vi "Demo.vi"() -> ()   [LabVIEW 2019]
uses:
  Components/MES_Base.lvlibp/Controls/Test.ctl
  Components/TestView_Base.lvlibp/ViewStatus.ctl
  Components/TestView_Base.lvlibp/TestView_Base.lvclass
  C:/Projects/Client-Nanosonics/Src/Components/ViPER.lvlibp/ViPER.lvclass
  Components/ViPER.lvlibp/ViPER.lvclass
  Components/MES_Base.lvlibp/MES_Base.lvclass
panel:
  in  "Exit":bool caption="Blank"
  out "error out":errorcluster
  in  "Clear":bool
  in  "DUT":u32
  in  "User":string
  in  "set User":bool
  in  "Status":T1
  in  "set status":bool
  in  "Test":T2={"Code"="", "Name"="", "Description"="", "Group"="", "IsGroup"=FALSE, "Tag"="", "Method"="", "Parrameter"="", "DataType"=enum."String", "Value"=variant, "Status"=enum."Pass", "LimitLo"=variant, "LimitHi"=variant, "StringMatch"="", "BooleanMatch"=FALSE, "DisplayFormat"="", "Units"="", "TestTime"=0.0}
  in  "Set test":bool
  in  "Tests":T2[](array[typedef])
  in  "Set tests":bool
  in  "Title":string
  in  "set title":bool
  in  "SN":string
  in  "set SN":bool
  in  "stop":bool
  in  "Config XML":string="<?xml version=\"1.0\" encoding=\"UTF-8\" standalone=\"no\" ?>\n<Object>\n\n  <Name>TestView</Name>\n\n  <Class>TestView_Bailey</Class>\n\n</Object>\n"
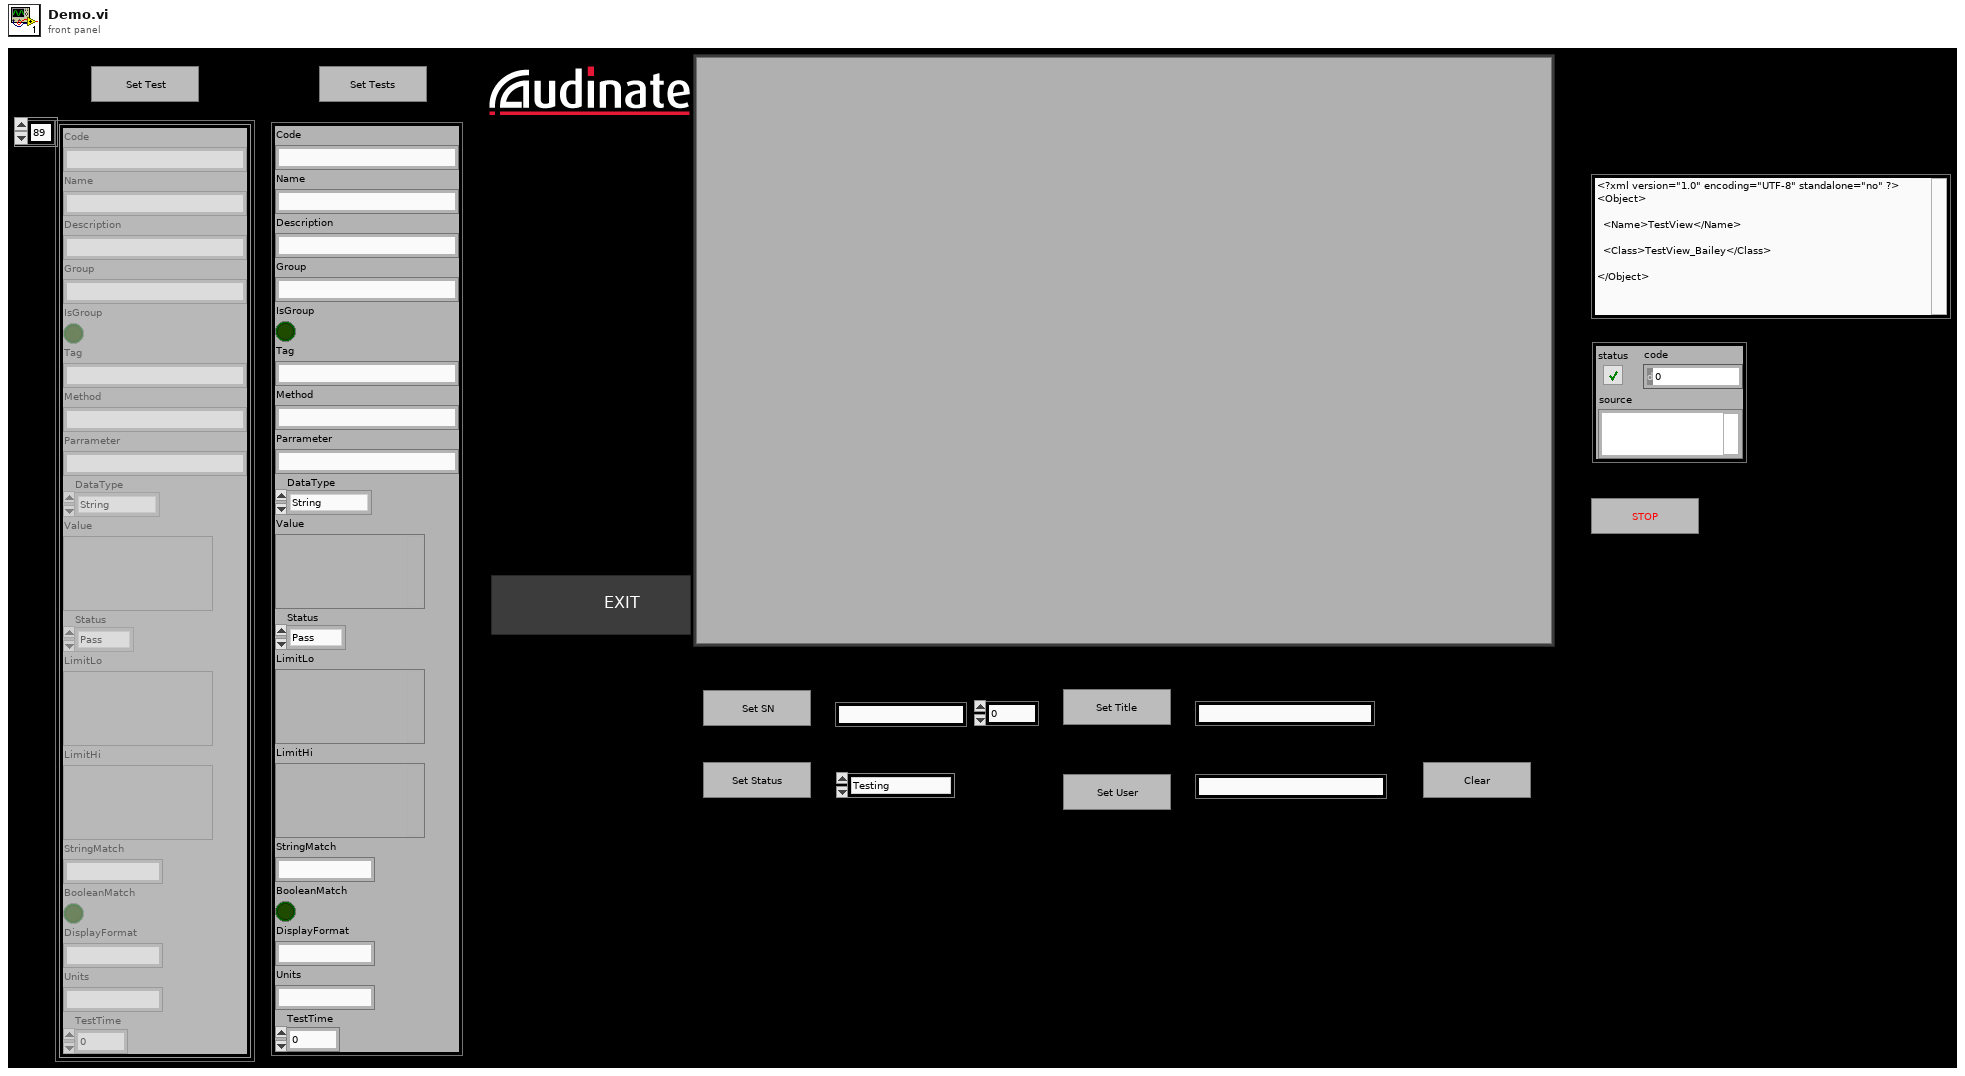
[diagram p1: front panel]
types:
  T1 = typedef "TestView_Base.lvlibp/TestView_Base.lvclass/ViewStatus.ctl" = enum16{"Testing", "Ready", "Logout", "Login", "PASS", "FAIL", "FAULT", "ABORTED"}
  T2 = typedef "MES_Base.lvlibp/MES_Base.lvclass/Test.ctl" = cluster{"Code":string, "Name":string, "Description":string, "Group":string, "IsGroup":bool, "Tag":string, "Method":string, "Parrameter":string, "DataType":enum16{"NA", "String", "Boolean", "Int", "Dbl"}, "Value":variant, "Status":enum16{"Pending", "Pass", "Fail"}, "LimitLo":variant, "LimitHi":variant, "StringMatch":string, "BooleanMatch":bool, "DisplayFormat":string, "Units":string, "TestTime":dbl}
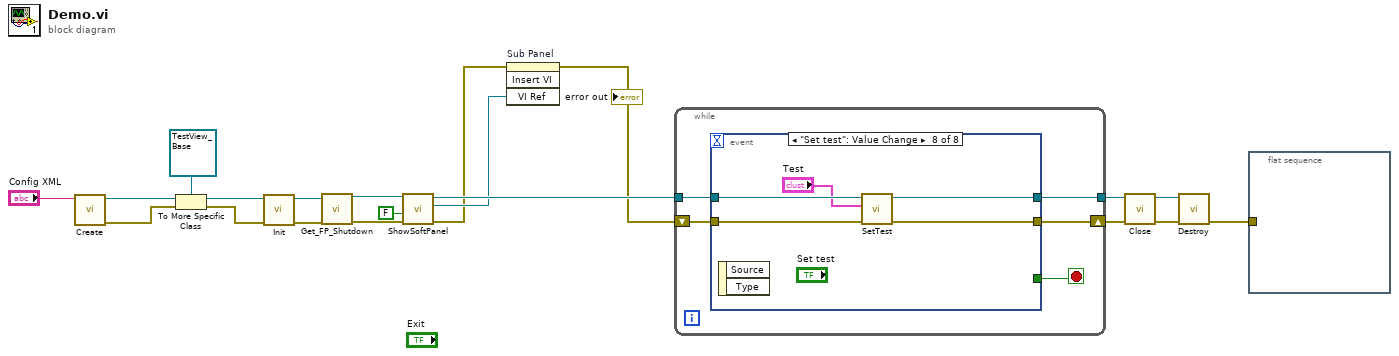
[diagram p0: block diagram]
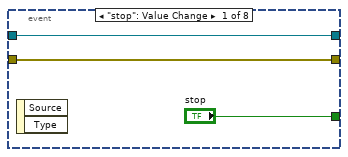
[diagram p2: hidden frame]
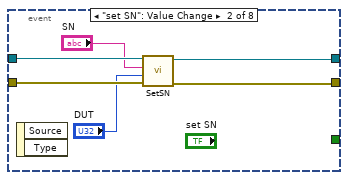
[diagram p3: hidden frame]
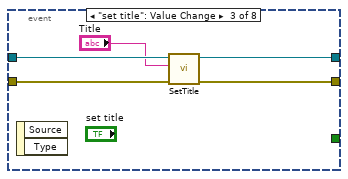
[diagram p4: hidden frame]
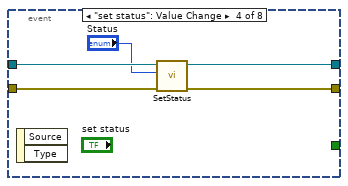
[diagram p5: hidden frame]
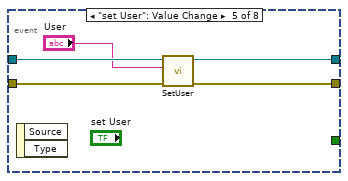
[diagram p6: hidden frame]
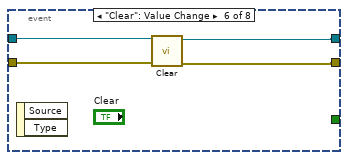
[diagram p7: hidden frame]
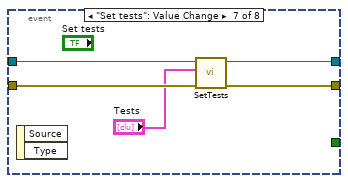
[diagram p8: hidden frame]
diagram:
  n1 = call "Create.vi"("Config XML"="Config XML") -> ("error out"=w9:errorcluster, "reference out"=w7:refnum<class "ViPER.lvclass">)  [unwired: 9 in]
  n2 = To More Specific Class(target class=refnum<class "TestView_Base.lvclass"> refnum ("TestView_Base.lvlibp:TestView_Tree"), reference=w7, error in=w9) -> (specific class reference=w6:refnum<class "TestView_Base.lvclass">, error out=w8:errorcluster)
  n3 = call-dynamic "Init.vi"("error in (no error)"=w8, "reference in"=w6) -> ("error out"=w19:errorcluster, "reference in"=w18:refnum<class "TestView_Base.lvclass">)  [unwired: 8 in]
  n4 = call "Get_FP_Shutdown.vi"("ViKing_Base in"=w18, "error in (no error)"=w19) -> ("ViKing_Base out"=w16:refnum<class "TestView_Base.lvclass">, "error out"=w17:errorcluster)  [unwired: 9 in, 3 out]
  n5 = call-dynamic "ShowSoftPanel.vi"("error in (no error)"=w17, "Floating"=FALSE, "Driver in"=w16) -> ("error out"=w2:errorcluster, "vi reference"=w3:refnum<vi>, "Driver out"=w5:refnum<class "TestView_Base.lvclass">)  [unwired: 6 in]
  n6 = invoke on="Sub Panel" class="SubPnl" method="Insert VI"(error in=w2, "VI Ref"=w3) -> (error out=w1:errorcluster)  [unwired: 2 in, 3 out]
  "error out" <- w1
  n7 = while {
    tunnel: w5 -> [w24]
    shift-right: [w22] -> w12
    shift-left: w1 -> [w25]
    tunnel: [w21] -> w13
    stop <- w23 stop-if-true
    n8 = event shown="[7] \"Set test\": Value Change" {
      selector: _ -> [_ _ _ _ _ _ _ _]
      dyn-events: _ -> [_ _ _ _ _ _ _ _]
      timeout: _ -> [_ _ _ _ _ _ _ _]
      tunnel: w25 -> [w27 w34 w39 w44 w49 w53 w58 w63]
      tunnel: w24 -> [w26 w33 w38 w43 w48 w52 w56 w62]
      tunnel: ["stop" _ _ _ _ _ _ _] -> w23
      tunnel: [w27 w32 w37 w42 w47 w51 w57 w61] -> w22
      tunnel: [w26 w31 w36 w41 w46 w50 w55 w60] -> w21
      event "stop": Value Change {
        n9 = event-data() -> ()  [unwired: 1 in, 2 out]
      }
      event "set SN": Value Change {
        n10 = event-data() -> ()  [unwired: 1 in, 2 out]
        n11 = call-dynamic "SetSN.vi"("error in (no error)"=w34, "DUT"="DUT", "SN"="SN", "reference in"=w33) -> ("error out"=w32:errorcluster, "reference in"=w31:refnum<class "TestView_Base.lvclass">)  [unwired: 6 in]
      }
      event "set title": Value Change {
        n12 = event-data() -> ()  [unwired: 1 in, 2 out]
        n13 = call-dynamic "SetTitle.vi"("error in (no error)"=w39, "Title"="Title", "reference in"=w38) -> ("error out"=w37:errorcluster, "reference in"=w36:refnum<class "TestView_Base.lvclass">)  [unwired: 7 in]
      }
      event "set status": Value Change {
        n14 = event-data() -> ()  [unwired: 1 in, 2 out]
        n15 = call-dynamic "SetStatus.vi"("error in (no error)"=w44, "Status"="Status", "reference in"=w43) -> ("error out"=w42:errorcluster, "reference in"=w41:refnum<class "TestView_Base.lvclass">)  [unwired: 7 in]
      }
      event "set User": Value Change {
        n16 = event-data() -> ()  [unwired: 1 in, 2 out]
        n17 = call-dynamic "SetUser.vi"("error in (no error)"=w49, "User"="User", "reference in"=w48) -> ("error out"=w47:errorcluster, "reference in"=w46:refnum<class "TestView_Base.lvclass">)  [unwired: 7 in]
      }
      event "Clear": Value Change {
        n18 = event-data() -> ()  [unwired: 1 in, 2 out]
        n19 = call-dynamic "Clear.vi"("error in (no error)"=w53, "TestView_Tree in"=w52) -> ("error out"=w51:errorcluster, "TestView_Tree out"=w50:refnum<class "TestView_Base.lvclass">)  [unwired: 8 in]
      }
      event "Set tests": Value Change {
        n20 = event-data() -> ()  [unwired: 1 in, 2 out]
        n21 = call-dynamic "SetTests.vi"("error in (no error)"=w58, "Tests"="Tests", "reference in"=w56) -> ("error out"=w57:errorcluster, "reference in"=w55:refnum<class "TestView_Base.lvclass">)  [unwired: 7 in]
      }
      event "Set test": Value Change {
        n22 = event-data() -> ()  [unwired: 1 in, 2 out]
        n23 = call-dynamic "SetTest.vi"("error in (no error)"=w63, "Test"="Test", "reference in"=w62) -> ("error out"=w61:errorcluster, "reference in"=w60:refnum<class "TestView_Base.lvclass">)  [unwired: 7 in]
      }
    }
  }
  n24 = call-dynamic "Close.vi"("error in (no error)"=w12, "reference in"=w13) -> ("error out"=w15:errorcluster, "reference in"=w14:refnum<class "TestView_Base.lvclass">)  [unwired: 8 in]
  n25 = call "Destroy.vi"("error in (no error)"=w15, "reference in"=w14) -> ("error out"=w4:errorcluster)  [unwired: 9 in]
  n26 = flat-sequence {
    tunnel: w4 -> [_]
    frame #0 {
    }
  }
